vi "ErrorControlMissing.vi"(0 "Create Error?":bool, 5 "Control Name":string, 11 "error in":errorcluster) -> (15 "error out":errorcluster)   [LabVIEW 2016, in "Drona.lvlib"]
doc: "Creates error if the control is not found."
uses:
  Drona.lvlib
  <vilib>/Utility/error.llb/Error Cluster From Error Code.vi
  <vilib>/ErrorRing/Error Ring.xnode
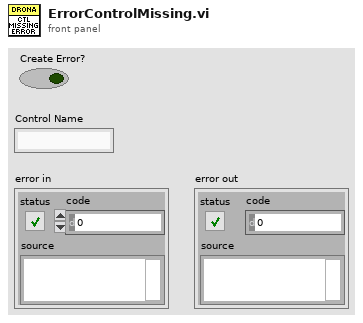
[diagram p1: front panel]
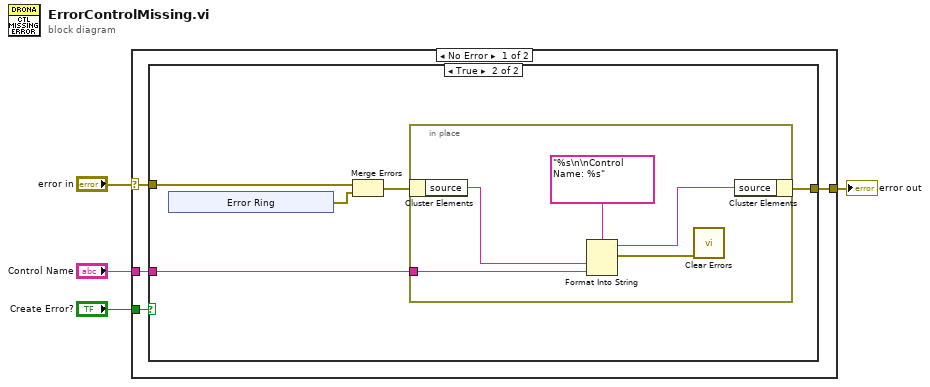
[diagram p0: block diagram]
diagram:
  n1 = case shown="No Error" "error in" {
    selector: "error in" -> [w5 w25]
    tunnel: "Control Name" -> [w8 _]
    tunnel: [w7 w25] -> w3
    tunnel: "Create Error?" -> [w6 _]
    frame No Error {
      n2 = case shown="True" w6 {
        tunnel: w5 -> [w9 w14]
        tunnel: [w9 w11] -> w7
        tunnel: w8 -> [_ w10]
        frame False {
        }
        frame True {
          n3 = xnode "Error Ring"() -> ("error out"=w13:errorcluster)
          n4 = Merge Errors(w14, w13) -> (w12:errorcluster)
          n5 = in-place {
            in-place-border: w10 -> [w19]
            n6 = in-place-cluster #1(w12) -> ("source"=w16:string)
            n7 = Format Into String(format string="%s\n\nControl Name: %s", w16, w19) -> (resulting string=w17:string, error out=w15:errorcluster)  [unwired: 2 in]
            n8 = call <vilib>:"Clear Errors.vi"("error in (no error)"=w15) -> ()  [unwired: 5 in, 2 out]
            n9 = in-place-cluster #1("source"=w17) -> (w11:errorcluster)
          }
        }
      }
    }
    frame Error {
    }
  }
  "error out" <- w3
